vi "Modules Catalog.vi"(8 "error in (no error)":errorcluster, 10 "Module":string, 11 "launcher in":refnum<class "launcher.lvclass">) -> (0 "error out":errorcluster, 1 "Selected Module":refnum<class "Module.lvclass">, 3 "launcher out":refnum<class "launcher.lvclass">)   [LabVIEW 2021, in "launcher.lvclass"]
uses:
  launcher.lvclass
  <userlib>/S2 Labs/Module Framework/Modules/Base/Module.lvclass
  Sim DiscreteIO/Sim DiscreteIO.lvclass
  C:/Program Files (x86)/National Instruments/LabVIEW 2021/user.lib/S2 Labs/Module Framework/Modules/Base/Module.lvclass
  Slave Modules/Battery Pack/Battery Pack.lvclass
  Formulas Module/Formulas Module.lvclass
  iC7-AFE/iC7-AFE.lvclass
  iC7-DCDC/iC7-DCDC.lvclass
  iC7-INU/iC7-INU.lvclass
  Vacon-DCGuard/Vacon-DCGuard.lvclass
  ComAp-Generator/ComAp-Generator.lvclass
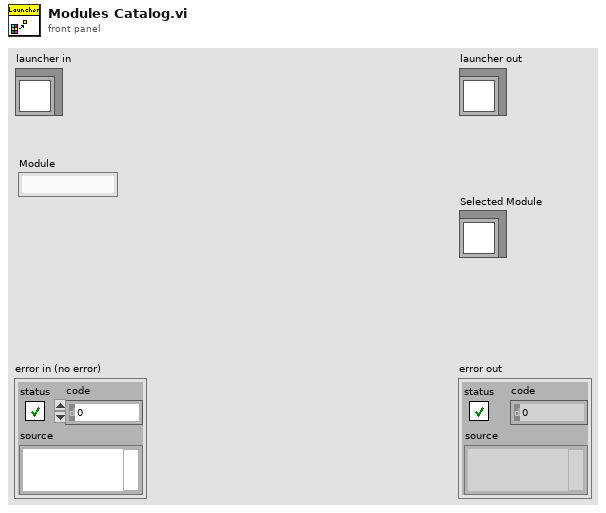
[diagram p1: front panel]
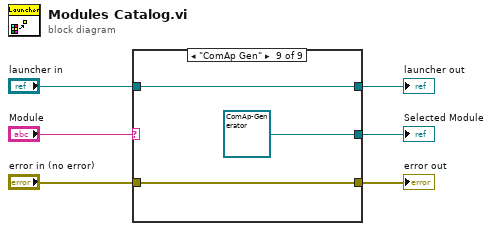
[diagram p0: block diagram]
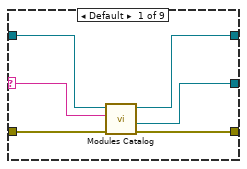
[diagram p2: hidden frame]
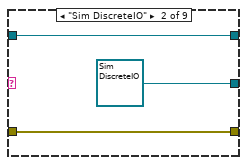
[diagram p3: hidden frame]
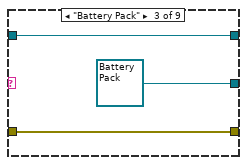
[diagram p4: hidden frame]
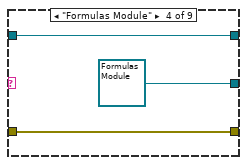
[diagram p5: hidden frame]
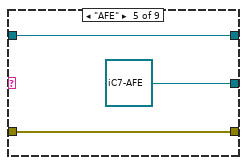
[diagram p6: hidden frame]
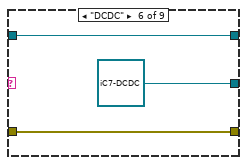
[diagram p7: hidden frame]
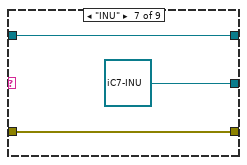
[diagram p8: hidden frame]
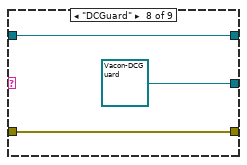
[diagram p9: hidden frame]
diagram:
  n1 = case shown="\"ComAp Gen\"" "Module" {
    selector: "Module" -> [w8 _ _ _ _ _ _ _ _]
    tunnel: [w12 w13 w18 w21 w22 w25 w28 w32 w34] -> w6
    tunnel: [w11 refnum<class "Sim DiscreteIO.lvclass"> refnum ("Sim DiscreteIO") refnum<class "Battery Pack.lvclass"> refnum ("Modbus Slave Module") refnum<class "Formulas Module.lvclass"> refnum ("Formulas Module") refnum<class "iC7-AFE.lvclass"> refnum ("iC7-AFE") refnum<class "iC7-DCDC.lvclass"> refnum ("iC7-DCDC") refnum<class "iC7-INU.lvclass"> refnum ("iC7-INU") refnum<class "Vacon-DCGuard.lvclass"> refnum ("Vacon-DCGuard") refnum<class "ComAp-Generator.lvclass"> refnum ("ComAp-Gen")] -> w5
    tunnel: [w10 w15 w17 w20 w24 w27 w29 w31 w36] -> w4
    tunnel: "error in (no error)" -> [w9 w13 w18 w21 w22 w25 w28 w32 w34]
    tunnel: "launcher in" -> [w7 w15 w17 w20 w24 w27 w29 w31 w36]
    frame Default {
      n2 = call-parent "Modules Catalog.vi"("error in (no error)"=w9, "Module"=w8, "Module in"=w7) -> ("error out"=w12:errorcluster, "Selected Module"=w11:refnum<class "Module.lvclass">, "Module out"=w10:refnum<class "launcher.lvclass">)  [unwired: 6 in]
    }
    frame "Sim DiscreteIO" {
    }
    frame "Battery Pack" {
    }
    frame "Formulas Module" {
    }
    frame "AFE" {
    }
    frame "DCDC" {
    }
    frame "INU" {
    }
    frame "DCGuard" {
    }
    frame "ComAp Gen" {
    }
  }
  "error out" <- w6
  "launcher out" <- w4
  "Selected Module" <- w5
